vi "add data to digestsign.vi"(8 "error in":errorcluster, 10 "data to add":string, 11 "lvlibcrypto digest in":refnum<class "lvlibcrypto digestsign.lvclass">) -> (0 "error out":errorcluster, 3 "lvlibcrypto digest out":refnum<class "lvlibcrypto digestsign.lvclass">)   [LabVIEW 2016, in "lvlibcrypto digestsign.lvclass"]
uses:
  lvlibcrypto digestsign.lvclass
  lvlibcrypto digestsign.lvclass/lvlibcrypto digestsign.ctl
  lv tls dll.lvlib
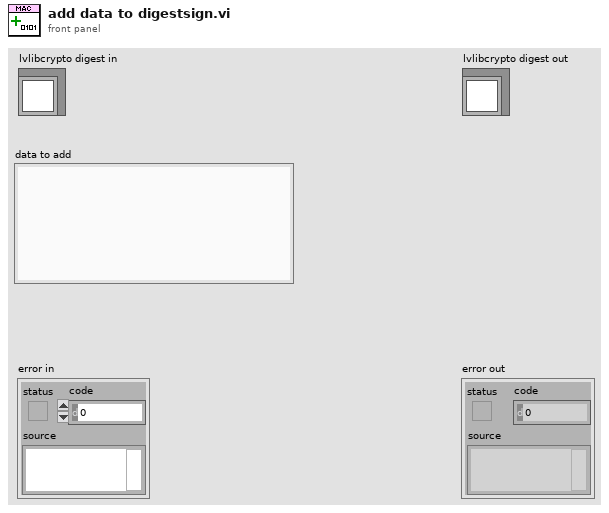
[diagram p1: front panel]
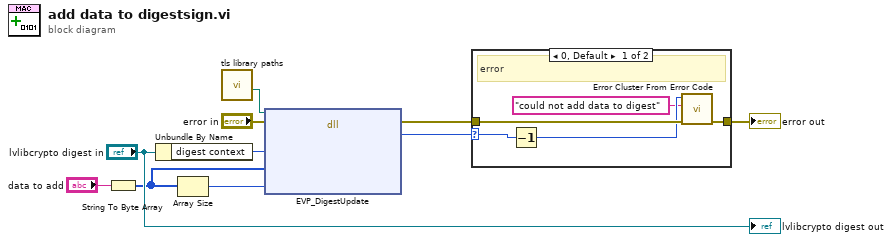
[diagram p0: block diagram]
diagram:
  n1 = String To Byte Array(string="data to add") -> (unsigned byte array=w2:u8[])
  n2 = Unbundle By Name("lvlibcrypto digest in") -> ("digest context"=w4:u64)
  n3 = Array Size(array=w2) -> (size(s)=w1:i32)
  n4 = call "tls library paths.vi"() -> ("libcrypto"=w9:path)  [unwired: 8 in, 3 out]
  n5 = dll-call lib="C:/Users/IEUser/Desktop/tlssimple/libcrypto-41.dll" fn="EVP_DigestUpdate"(path in=w9, error in="error in", "context"=w4, "data"=w2, "size"=w1) -> (error out=w5:errorcluster, "ret"=w6:i32)  [unwired: 4 in, 1 out]
  n6 = case shown="0, Default" w6 {
    selector: w6 -> [w13 _]
    tunnel: [w14 w16] -> w8
    tunnel: w5 -> [w15 w16]
    frame 0, Default {
      # "error"
      n7 = Decrement(x=w13) -> (x-1=w12:i32)
      n8 = call <vilib>:"Error Cluster From Error Code.vi"("error in (no error)"=w15, "error message (\"\")"="could not add data to digest" ("error message (\"\")"), "error code (0)"=w12) -> ("error out"=w14:errorcluster)  [unwired: 6 in]
    }
    frame 1 {
      # "success"
    }
  }
  "error out" <- w8
  "lvlibcrypto digest out" <- "lvlibcrypto digest in"
